vi "combine-info-to-cmd.vi"(9 "值":string="06102", 10 "寄存器":string="06102", 11 "info":T1) -> (3 "command":string)   [LabVIEW 2019]
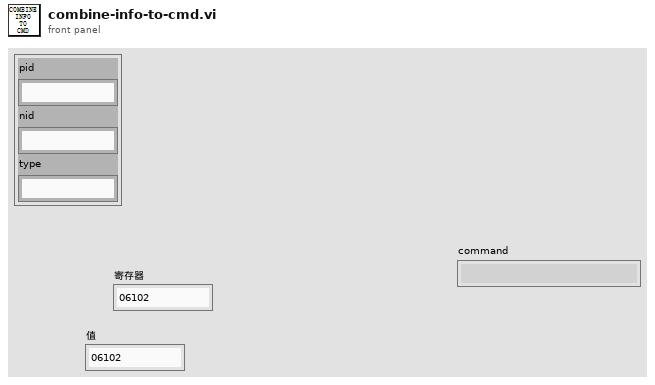
[diagram p1: front panel]
types:
  T1 = cluster{"pid":string, "nid":string, "type":string}
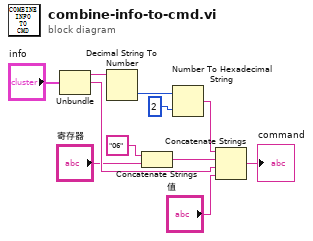
[diagram p0: block diagram]
diagram:
  n1 = Unbundle("info") -> ("pid"=w8:string, "nid"=w11:string)  [unwired: 1 out]
  n2 = Decimal String To Number(string=w8) -> (number=w1:i32)  [unwired: 2 in, 1 out]
  n3 = Concatenate Strings("06" ("字符串"), "寄存器") -> (w6:string)
  n4 = Number To Hexadecimal String(1:i16 2 ("宽度(-)"), 2:w1) -> (0:w10:string)
  n5 = Concatenate Strings(w10, w6, w11, "值") -> (→"command":string)
